vi "SafetySystem.vi"() -> ()   [LabVIEW 2018]
uses:
  <vilib>/Platform/TimedLoop/XDataNode/timing_clust.ctl
  <vilib>/Platform/TimedLoop/XDataNode/nitl_modes.ctl
  <vilib>/Platform/TimedLoop/XDataNode/wakeup.ctl
  <vilib>/myRIO/Common/Instrument Driver Framework/myRIO v1.0/UART/vis/myRIO v1.0 Close UART.vi
  <vilib>/Modbus/slave/Create Slave Instance (TCP).vi
  <vilib>/myRIO/Common/Instrument Driver Framework/Utilities/vis/FPGA Ref Manager.vi
  <vilib>/myRIO/Common/Instrument Driver Framework/myRIO v1.0/myRIO v1.0 Reset FPGA.vi
  <vilib>/myRIO/Common/Instrument Driver Framework/myRIO v1.0/IRQ/vis/myRIO v1.0 IRQ Info FGV.vi
  <vilib>/myRIO/Common/Instrument Driver Framework/myRIO v1.0/IRQ/vis/myRIO v1.0 Timer IRQ Info FGV.vi
  <vilib>/myRIO/Common/Instrument Driver Framework/myRIO v1.0/IRQ/vis/myRIO v1.0 ISR Agent.vi
  <vilib>/Modbus/slave/Modbus Slave.lvclass
  <vilib>/Platform/TimedLoop/XDataNode/XDataNode.xnode
  <vilib>/Platform/TimedLoop/XDataNode/XDNodeRunTimeDep.lvlib
  <vilib>/myRIO/Instrument Drivers/Utilities/Utilities.lvlib
panel:
  out "error out":errorcluster
  out "TX-SIS-BPCS-ARRAY":bool[](array[boolean])
  out "SIS-10SDV501":bool
  out "SIS-10SDV502":bool
  out "SIS-10SDV500":bool
  out "SIS-10TI101":dbl
  out "SIS-10AI301":dbl
  out "SIS-10LI202":dbl
  out "SIS-10LI201":dbl
  in  "stop":bool
  out "SIS-SIM-TX-ARRAY":dbl[](array[numeric])
  out "SIM-SIS-RX-ARRAY":dbl[](array[numeric])
  # "SIS-10SDV502"
  # "SIS-10LI201"
  # "SIS-10SDV500"
  # "SIS-10SDV501"
  # "SIS-10LI202"
  # "SIS-10AI301"
  # "SIS-10TI101"
  # "SIS-10SDV500"
  # "SIS-10SDV501"
  # "SIS-10SDV502"
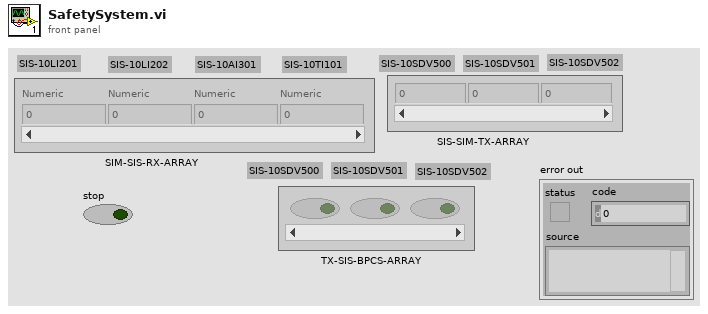
[diagram p1: front panel]
types:
  T1 = typedef "XDNodeRunTimeDep.lvlib/timing_clust.ctl" = cluster{"Expected End [f-1]":u64, "Actual End [f-1]":u64, "Finished Late? [f-1]":bool, "Expected End [i-1]":u64, "Actual End [i-1]":u64, "Finished Late? [i-1]":bool, "Expected Start [i]":u64, "Actual Start [i]":u64, "Expected Start [f]":u64, "Actual Start [f]":u64, "Source Name":string, "Structure Name":string, "Period":i64, "Deadline":i64, "Offset":i64, "Start":i64, "Priority":i32, "Timeout":i32, "Mode":T2, "Wakeup Reason":T3, "Error":errorcluster, "Source Type":string, "Secondary Source Type":string, "Global End Time":u64, "Global Start Time":u64, "Frame Duration":u64, "Iteration Duration":u64, "Assigned CPU":i32, "I/O Scan Engine Mode":u32}
  T2 = typedef "XDNodeRunTimeDep.lvlib/nitl_modes.ctl" = enum32{"No Change", "Process missed periods, maintain original phase", "Discard missed periods, maintain original phase", "Process missed periods, ignore original phase", "Discard missed periods, ignore original phase"}
  T3 = typedef "XDNodeRunTimeDep.lvlib/wakeup.ctl" = enum32{"Normal", "Aborted", "Asynchronous wakeup", "Timing source error", "Timed loop error", "Timeout"}
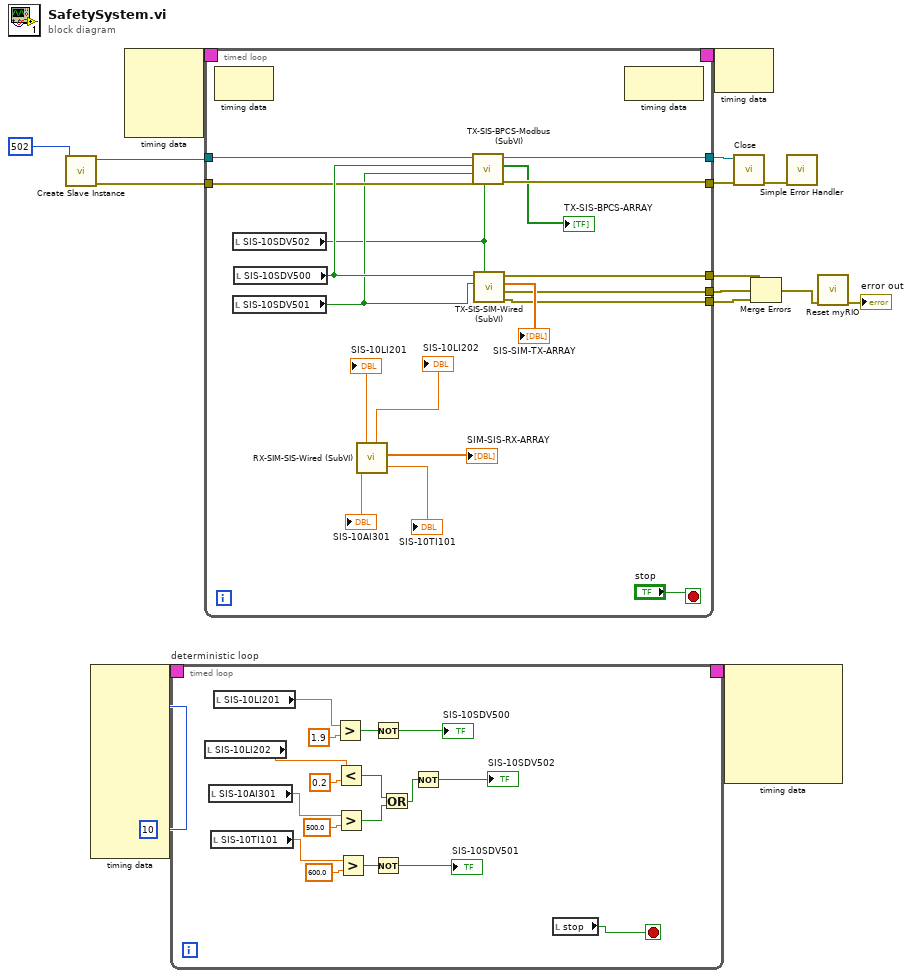
[diagram p0: block diagram]
diagram:
  n1 = call-poly <vilib>:"Create Slave Instance.vi"("port (502)"=u16 502) -> ("error out"=w10:errorcluster, "TCP slave instance"=w11:refnum<class "Modbus Slave.lvclass">)  [unwired: 9 in]
  n2 = node-c288 ("Input Node")(i64 10 ("Period")) -> (w16:T1)  [unwired: 9 in]
  n3 = node-c288() -> (w13:T1)  [unwired: 4 in]
  n4 = timed-loop "deterministic loop" {
    timing: w16 -> [_]
    timing-out: [_] -> w15
    stop <- w20 stop-if-true
    n5 = local read "SIS-10LI202"() -> (w26:dbl)
    n6 = local read "SIS-10AI301"() -> (w25:dbl)
    n7 = local read "SIS-10TI101"() -> (w24:dbl)
    n8 = local read "SIS-10LI201"() -> (w27:dbl)
    n9 = Greater?(x=w27, y=1.9) -> (0:w32:bool)
    n10 = Less?(x=w26, y=0.2) -> (x < y?=w18:bool)
    n11 = Greater?(x=w25, y=500.0) -> (0:w19:bool)
    n12 = Greater?(x=w24, y=600.0) -> (0:w30:bool)
    n13 = Not(x=w32) -> (.not. x?=→"SIS-10SDV500":bool)
    n14 = Not(x=w30) -> (.not. x?=→"SIS-10SDV501":bool)
    n15 = Or(x=w18, y=w19) -> (x .or. y?=w17:bool)
    n16 = Not(x=w17) -> (.not. x?=→"SIS-10SDV502":bool)
    n17 = local read "stop"() -> (w20:bool)
  }
  n18 = timed-loop {
    timing: w13 -> [_]
    timing-out: [_] -> w12
    tunnel: w11 -> [w49]
    tunnel: [w48] -> w8
    tunnel: w10 -> [w44]
    tunnel: [w47] -> w7
    tunnel: [w38] -> w5
    tunnel: [w37] -> w4
    tunnel: [w36] -> w3
    stop <- "stop" stop-if-true
    n19 = node-c288() -> ()  [unwired: 1 in, 1 out]
    n20 = local read "SIS-10SDV502"() -> (w40:bool)
    n21 = local read "SIS-10SDV501"() -> (w41:bool)
    n22 = local read "SIS-10SDV500"() -> (w45:bool)
    n23 = call "RX-SIM-SIS-Wired (SubVI).vi"() -> ("SIM-SIS-RX-ARRAY"=→"SIM-SIS-RX-ARRAY":dbl[], "SIS-10TI101"=→"SIS-10TI101":dbl, "SIS-10LI202"=→"SIS-10LI202":dbl, "SIS-10AI301"=→"SIS-10AI301":dbl, "SIS-10LI201"=→"SIS-10LI201":dbl)  [unwired: 7 in]
    n24 = call "TX-SIS-BPCS-Modbus (SubVI).vi"("SIS-10SDV502"=w40, "error in (no error)"=w44, "SIS-10SDV501"=w41, "SIS-10SDV500"=w45, "Modbus Slave in"=w49) -> ("error out"=w47:errorcluster, "TX-SIS-BPCS-ARRAY"=→"TX-SIS-BPCS-ARRAY":bool[], "Modbus Slave out"=w48:refnum<class "Modbus Slave.lvclass">)  [unwired: 4 in]
    n25 = call "TX-SIS-SIM-Wired (SubVI).vi"("SIS-10SDV502"=w40, "SIS-10SDV501"=w41, "SIS-10SDV500"=w45) -> ("error out 3"=w36:errorcluster, "error out 2"=w37:errorcluster, "SIS-SIM-TX-ARRAY"=→"SIS-SIM-TX-ARRAY":dbl[], "error out"=w38:errorcluster)  [unwired: 5 in]
    n26 = node-c288() -> ()  [unwired: 1 in, 1 out]
  }
  n27 = node-c288(w12) -> ()  [unwired: 1 out]
  n28 = node-c288 ("Output Node")(w15) -> ()  [unwired: 6 out]
  n29 = call-dynamic "Close.vi"("error in (no error)"=w7, "Modbus slave in"=w8) -> ("error out"=w9:errorcluster)  [unwired: 9 in]
  n30 = Merge Errors(w5, w4, w3) -> (w2:errorcluster)
  n31 = call <vilib>:"Simple Error Handler.vi"("error in (no error)"=w9) -> ()  [unwired: 4 in, 5 out]
  n32 = call <vilib>:"Reset myRIO.vi"("error in (no error)"=w2) -> ("error out"=→"error out":errorcluster)  [unwired: 10 in]
